vi "Init Frame Grabber.vi"(6 "Frame Grabber":T2="cam1", 8 "Error In":errorcluster, 11 "Frame Grabber Data In":T1={"Camera Session"="", "Frame"=refnum, "AVI Refnum"=refnum, "Codecs"=[], "Frame number"=0, "Tracking File Refnum"=refnum, "Tick Count"=0, "Probe Object"=refnum, "Playback Probe Data"=[], "Rigid Body"={"Position"={"x (mm)"=0.0, "y (mm)"=0.0, "z (mm)"=0.0}, "Orientation"={"Pitch (rad)"=0.0, "Yaw (rad)"=0.0, "Roll (rad)"=0.0}, "Quaternion"={"qx"=0.0, "qy"=0.0, "qz"=0.0, "qw"=0.0}, "Tracked?"=FALSE}, "Total no frames playback"=0, "Video FPS"=0.0, "Camera connected?"=FALSE, "Scene"=refnum, "Cropped Frame"=refnum, "Tracker FPS"=0.0, "Crop ROI"=[], "Presentation Values"=[], "Elapsed time (ms)"=0, "Camera frames playback"=0, "Refnums"={"Live Refnum"=refnum, "Record Refnum"=refnum, "Recording Settings Refnum"=refnum, "Playback Refnum"=refnum, "Frame Slider Refnum"=refnum, "Pause Refnum"=refnum, "Home Refnum"=refnum, "Crop Refnum"=refnum, "Clear Crop Refnum"=refnum, "stop refnum"=refnum, "Playback Rate Refnum"=refnum, "Operator Settings Refnums"=refnum, "Presentation Refnum"=refnum, "Gestation Refnum"=refnum, "Connection Settings Refnum"=refnum, "Crop Time Frame Slider Refnum"=refnum, "Cancel Save Refnum"=refnum, "Reverse Playback Refnum"=refnum}, "Dimensions"={"Probe Dimensions"={"Probe Width"=0.0, "Probe Depth"=1.0, "Probe Height"=0.0}, "Room Dimensions"={"Room Width"=0.0, "Room Depth"=0.0, "Room Height"=0.0}}, "Playback Data As Strings"=[], "Cropped Tracking File Refnum"=refnum, "Cropped AVI Refnum"=refnum, "Header"=[], "Total euclidian distance"=0.0, "Annotation File Path"=path "", "Playback File Path"=path ""}) -> (0 "Error Out":errorcluster={"status"=TRUE, "code"=1088, "source"="Property Node (arg 2) in NI_3D Picture Control.lvlib:Create Box.vi->Create 3D Shapes.vi->Init Frame Grabber.vi->Main.vi"}, 1 "Codec Names":string[](array[string])=["Cinepak Codec by Radius", "Intel IYUV codec", "Microsoft Video 1", "FF Video Codec 1 (FFV1) (NI Vision)", "Motion JPEG (NI Vision)", "Y800 Uncompressed Grey Scale (NI Vision)", "YUV 4:2:0 Planar (NI Vision)"], 2 "Frame Grabber Connected?":bool, 3 "Frame Grabber Data Out":T1={"Camera Session"="", "Frame"=refnum, "AVI Refnum"=refnum, "Codecs"=[], "Frame number"=0, "Tracking File Refnum"=refnum, "Tick Count"=0, "Probe Object"=refnum, "Playback Probe Data"=[], "Rigid Body"={"Position"={"x (mm)"=0.0, "y (mm)"=0.0, "z (mm)"=0.0}, "Orientation"={"Pitch (rad)"=0.0, "Yaw (rad)"=0.0, "Roll (rad)"=0.0}, "Quaternion"={"qx"=0.0, "qy"=0.0, "qz"=0.0, "qw"=0.0}, "Tracked?"=FALSE}, "Total no frames playback"=0, "Video FPS"=0.0, "Camera connected?"=FALSE, "Scene"=refnum, "Cropped Frame"=refnum, "Tracker FPS"=0.0, "Crop ROI"=[], "Presentation Values"=[], "Elapsed time (ms)"=0, "Camera frames playback"=0, "Refnums"={"Live Refnum"=refnum, "Record Refnum"=refnum, "Recording Settings Refnum"=refnum, "Playback Refnum"=refnum, "Frame Slider Refnum"=refnum, "Pause Refnum"=refnum, "Home Refnum"=refnum, "Crop Refnum"=refnum, "Clear Crop Refnum"=refnum, "stop refnum"=refnum, "Playback Rate Refnum"=refnum, "Operator Settings Refnums"=refnum, "Presentation Refnum"=refnum, "Gestation Refnum"=refnum, "Connection Settings Refnum"=refnum, "Crop Time Frame Slider Refnum"=refnum, "Cancel Save Refnum"=refnum, "Reverse Playback Refnum"=refnum}, "Dimensions"={"Probe Dimensions"={"Probe Width"=0.0, "Probe Depth"=1.0, "Probe Height"=0.0}, "Room Dimensions"={"Room Width"=0.0, "Room Depth"=0.0, "Room Height"=0.0}}, "Playback Data As Strings"=[], "Cropped Tracking File Refnum"=refnum, "Cropped AVI Refnum"=refnum, "Header"=[], "Total euclidian distance"=0.0, "Annotation File Path"=path "", "Playback File Path"=path ""}, 4 "Image Out":T3)   [LabVIEW 2017]
uses:
  <vilib>/userdefined/High Color/IMAQdx.ctl
  Controls/Frame Grabber Data.ctl
  <vilib>/vision/Image Controls.llb/IMAQ Image.ctl
  <vilib>/vision/Avi.llb/IMAQ AVI2 Refnum.ctl
  Controls/Rigid Body Info.ctl
  Controls/Position.ctl
  Controls/Orientation.ctl
  Controls/Refnums.ctl
  Controls/Recording Settings.ctl
  Controls/Operator Settings.ctl
  Controls/Operator.ctl
  Controls/Dimensions.ctl
  Controls/Room Dimensions.ctl
  <vilib>/vision/driver/IMAQdx.llb/IMAQdx Camera Control Mode.ctl
  <vilib>/vision/driver/NI_Vision_Acquisition_Software.lvlib
  <vilib>/vision/NI_Vision_Development_Module.lvlib
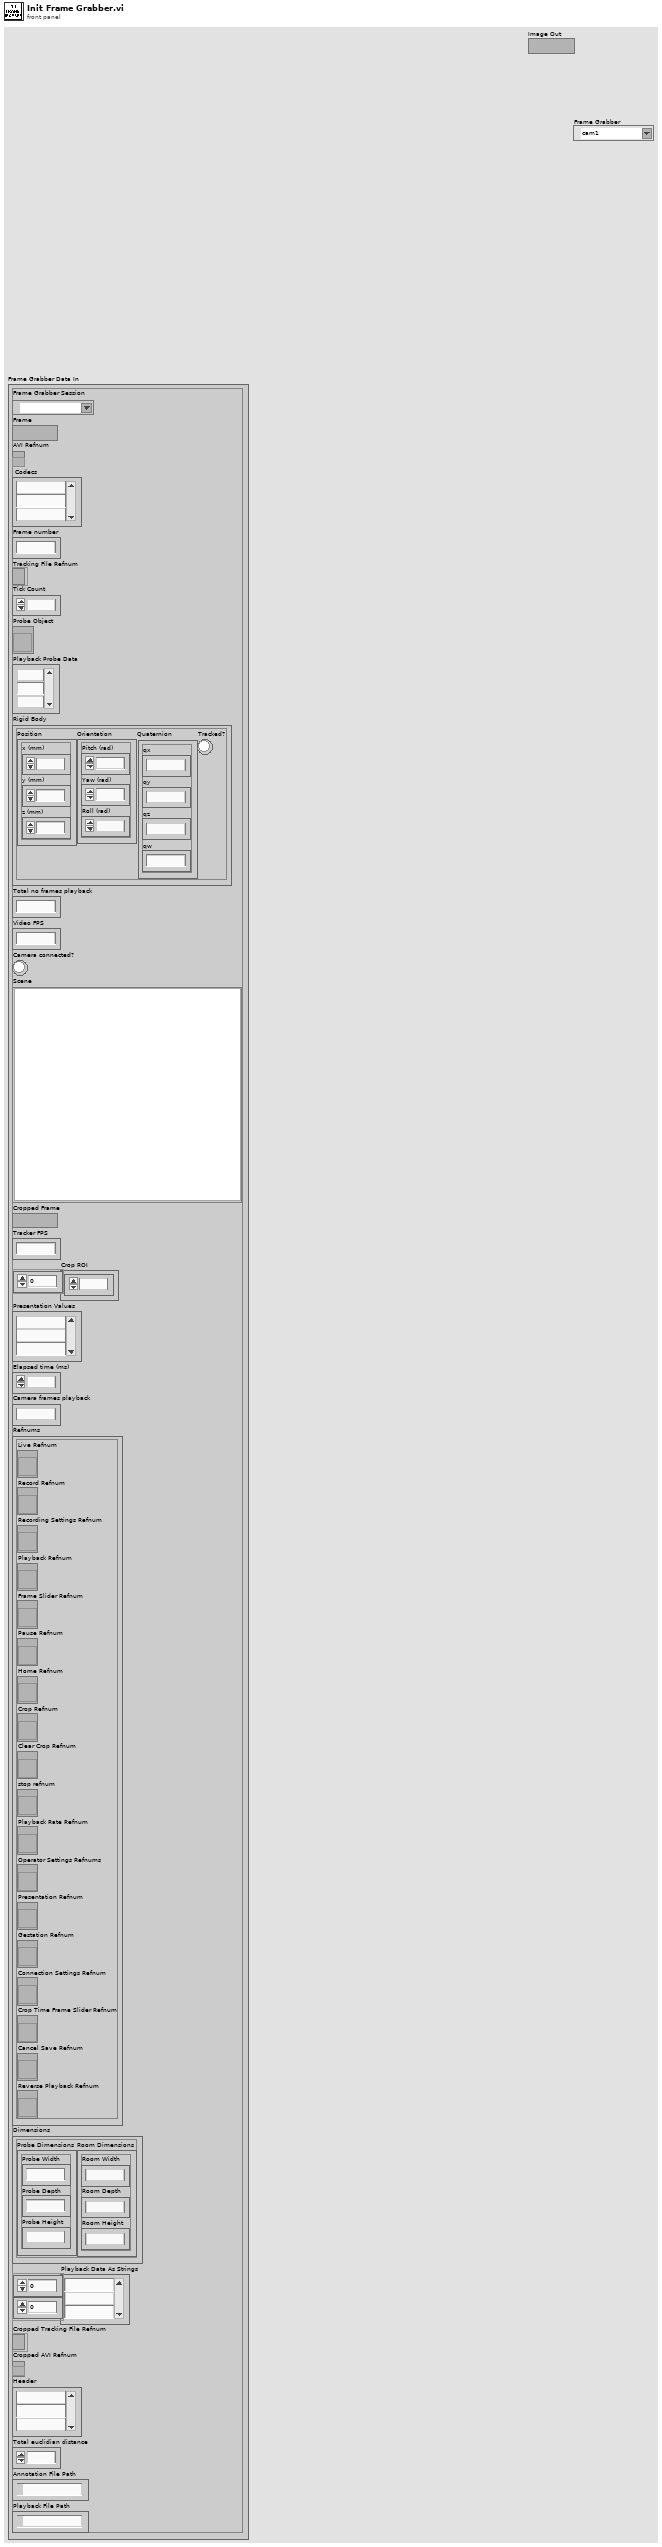
[diagram p1: front panel]
types:
  T1 = typedef "Frame Grabber Data.ctl" = cluster{"Camera Session":T2, "Frame":T3, "AVI Refnum":T4, "Codecs":string[], "Frame number":u32, "Tracking File Refnum":refnum<file>, "Tick Count":u32, "Probe Object":refnum<vi>, "Playback Probe Data":dbl[][], "Rigid Body":T5, "Total no frames playback":i32, "Video FPS":dbl, "Camera connected?":bool, "Scene":refnum<vi>, "Cropped Frame":T3, "Tracker FPS":dbl, "Crop ROI":i32[], "Presentation Values":string[], "Elapsed time (ms)":u32, "Camera frames playback":u32, "Refnums":T8, "Dimensions":T9, "Playback Data As Strings":string[][], "Cropped Tracking File Refnum":refnum<file>, "Cropped AVI Refnum":T4, "Header":string[], "Total euclidian distance":dbl, "Annotation File Path":path, "Playback File Path":path}
  T2 = typedef "IMAQdx.ctl" = refnum<k21>
  T3 = typedef "IMAQ Image.ctl" = refnum<image>
  T4 = typedef "IMAQ AVI2 Refnum.ctl" = refnum<k20>
  T5 = typedef "Rigid Body Info.ctl" = cluster{"Position":T6, "Orientation":T7, "Quaternion":cluster{"qx":sgl, "qy":sgl, "qz":sgl, "qw":sgl}, "Tracked?":bool}
  T6 = typedef "Position.ctl" = cluster{"x (mm)":sgl, "y (mm)":sgl, "z (mm)":sgl}
  T7 = typedef "Orientation.ctl" = cluster{"Pitch (rad)":sgl, "Yaw (rad)":sgl, "Roll (rad)":sgl}
  T8 = typedef "Refnums.ctl" = cluster{"Live Refnum":refnum<vi>, "Record Refnum":refnum<vi>, "Recording Settings Refnum":refnum<vi>, "Playback Refnum":refnum<vi>, "Frame Slider Refnum":refnum<vi>, "Pause Refnum":refnum<vi>, "Home Refnum":refnum<vi>, "Crop Refnum":refnum<vi>, "Clear Crop Refnum":refnum<vi>, "stop refnum":refnum<vi>, "Playback Rate Refnum":refnum<vi>, "Operator Settings Refnums":refnum<vi>, "Presentation Refnum":refnum<vi>, "Gestation Refnum":refnum<vi>, "Connection Settings Refnum":refnum<vi>, "Crop Time Frame Slider Refnum":refnum<vi>, "Cancel Save Refnum":refnum<vi>, "Reverse Playback Refnum":refnum<vi>}
  T9 = typedef "Dimensions.ctl" = cluster{"Probe Dimensions":cluster{"Probe Width":sgl, "Probe Depth":sgl, "Probe Height":sgl}, "Room Dimensions":T10}
  T10 = typedef "Room Dimensions.ctl" = cluster{"Room Width":dbl, "Room Depth":dbl, "Room Height":dbl}
  T11 = typedef "NI_Vision_Acquisition_Software.lvlib/IMAQdx Camera Control Mode.ctl" = enum32{"Controller", "Listener"}
  T12 = typedef "Image Type" = u32
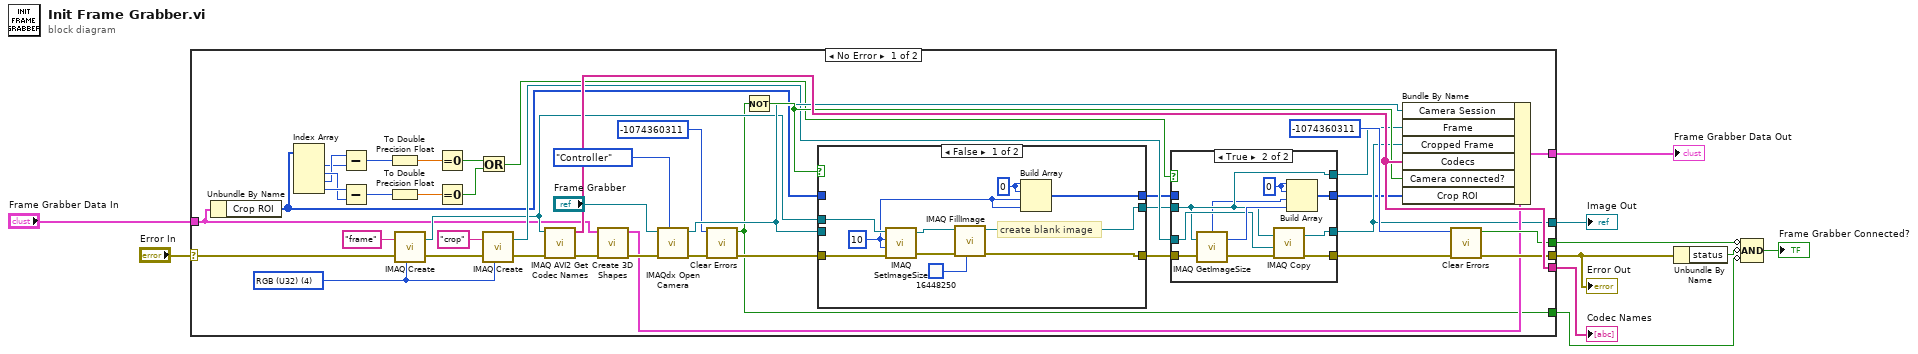
[diagram p0: block diagram]
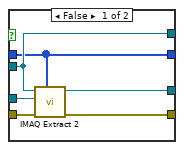
[diagram p2: hidden frame]
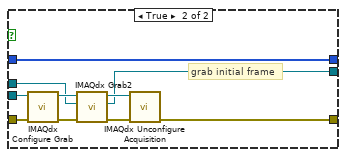
[diagram p3: hidden frame]
diagram:
  n1 = case shown="No Error" "Error In" {
    selector: "Error In" -> [w48 w91]
    tunnel: [w53 _] -> w4
    tunnel: [w45 w91] -> w9
    tunnel: [w51 _] -> w8
    tunnel: [w44 _] -> w6
    tunnel: [w24 _] -> w3
    tunnel: [w13 _] -> w2
    tunnel: "Frame Grabber Data In" -> [w12 _]
    frame No Error {
      w41 = T12 4 items=["Grayscale (U8)", "Grayscale (I16)", "Grayscale (SGL)", "Complex (CSG)", "RGB (U32)", "HSL (U32)", "RGB (U64)", "Grayscale (U16)"] ("Image Type")
      n2 = Unbundle By Name(w12) -> ("Crop ROI"=w11:i32[])
      n3 = Index Array(array=w11) -> (element #1=w19:i32, element #2=w21:i32, element #3=w20:i32, element #4=w22:i32)  [unwired: 4 in]
      n4 = Subtract(x=w20, y=w19) -> (x-y=w36:i32)
      n5 = Subtract(x=w22, y=w21) -> (x-y=w35:i32)
      n6 = To Double Precision Float(number=w36) -> (double precision float=w29:dbl)
      n7 = To Double Precision Float(number=w35) -> (double precision float=w28:dbl)
      n8 = call "IMAQ Create"("Image Name"="frame", "Image Type"=w41, "error in (no error)"=w48) -> ("New Image"=w26:T3, "error out"=w40:errorcluster)  [unwired: 2 in]
      n9 = Equal To 0?(x=w29) -> (x = 0?=w33:bool)
      n10 = Equal To 0?(x=w28) -> (x = 0?=w34:bool)
      n11 = Or(x=w33, y=w34) -> (x .or. y?=w32:bool)
      n12 = call "IMAQ Create"("Image Name"="crop", "Image Type"=w41, "error in (no error)"=w40) -> ("New Image"=w27:T3, "error out"=w39:errorcluster)  [unwired: 2 in]
      n13 = call "IMAQ AVI2 Get Codec Names"("error in (no error)"=w39, "Image"=w26) -> ("error out"=w49:errorcluster, "Codec Names"=w51:string[])  [unwired: 8 in]
      n14 = call "Create 3D Shapes.vi"("error in (no error)"=w49, "Frame Grabber Data In"=w12) -> ("error out"=w47:errorcluster, "Frame Grabber Data Out"=w43:T1)  [unwired: 8 in]
      n15 = call <vilib>:"IMAQdx Open Camera.vi"("Camera Control Mode"=IMAQdx_Camera_Control_Mode."Controller", "error in"=w47, "Session In"="Frame Grabber") -> ("error out"=w15:errorcluster, "Session Out"=w37:T2)  [unwired: 7 in]
      n16 = call <vilib>:"Clear Errors.vi"("error in (no error)"=w15, "specific error code to clear (0: all)"=-1074360311) -> ("error out"=w14:errorcluster, "specific error cleared?"=w13:bool)  [unwired: 4 in]
      n17 = Not(x=w13) -> (.not. x?=w38:bool)
      n18 = case shown="False" w38 {
        tunnel: w14 -> [w80 w87]
        tunnel: [w78 w86] -> w31
        tunnel: w37 -> [_ w85]
        tunnel: w26 -> [w77 w83]
        tunnel: [w75 w82] -> w25
        tunnel: w11 -> [_ w81]
        tunnel: [w73 w81] -> w17
        frame False {
          w72 = 0 ("element")
          w71 = 10 ("X Resolution")
          # "create blank image"
          n19 = call "IMAQ SetImageSize"("error in (no error)"=w80, "Y Resolution"=w71, "X Resolution"=w71, "Image"=w77) -> ("error out"=w79:errorcluster, "Image Out"=w76:T3)  [unwired: 1 in]
          n20 = call "IMAQ FillImage"("Color Pixel Value"=u32 16448250, "error in (no error)"=w79, "Image"=w76) -> ("error out"=w78:errorcluster, "Image Out"=w75:T3)  [unwired: 7 in]
          n21 = Build Array(w72, w72, w71, w71) -> (w73:i32[])
        }
        frame True {
          # "grab initial frame"
          n22 = call <vilib>:"IMAQdx Configure Grab.vi"("error in"=w87, "Session In"=w85) -> ("error out"=w88:errorcluster, "Session Out"=w90:T2)  [unwired: 8 in]
          n23 = call <vilib>:"IMAQdx Grab2.vi"("error in"=w88, "Image In"=w83, "Session In"=w90) -> ("error out"=w89:errorcluster, "Image Out"=w82:T3, "Session Out"=w84:T2)  [unwired: 5 in, 1 out]
          n24 = call <vilib>:"IMAQdx Unconfigure Acquisition.vi"("error in"=w89, "Session In"=w84) -> ("error out"=w86:errorcluster)  [unwired: 8 in, 1 out]
        }
      }
      n25 = case shown="True" w32 {
        tunnel: w25 -> [w56 w65]
        tunnel: w31 -> [w59 w69]
        tunnel: [w58 w64] -> w30
        tunnel: w27 -> [w60 w68]
        tunnel: w17 -> [w55 _]
        tunnel: [w56 w65] -> w23
        tunnel: [w57 w66] -> w24
        tunnel: [w55 w63] -> w18
        frame False {
          n26 = call "IMAQ Extract 2"("Optional Rectangle"=w55, "error in (no error)"=w59, "Image Dst"=w60, "Image Src"=w56) -> ("error out"=w58:errorcluster, "Image Dst Out"=w57:T3)  [unwired: 6 in]
        }
        frame True {
          w61 = 0 ("element")
          n27 = call "IMAQ GetImageSize"("Image"=w65, "error in (no error)"=w69) -> ("Y Resolution"=w70:i32, "X Resolution"=w62:i32, "error out"=w67:errorcluster)  [unwired: 2 in]
          n28 = call "IMAQ Copy"("error in (no error)"=w67, "Image Dst"=w68, "Image Src"=w65) -> ("error out"=w64:errorcluster, "Image Dst Out"=w66:T3)  [unwired: 3 in]
          n29 = Build Array(w61, w61, w62, w70) -> (w63:i32[])
        }
      }
      n30 = Bundle By Name(cluster=w43, "Camera Session"=w37, "Frame"=w23, "Cropped Frame"=w24, "Codecs"=w51, "Camera connected?"=w38, "Crop ROI"=w18) -> (w53:T1)
      n31 = call <vilib>:"Clear Errors.vi"("error in (no error)"=w30, "specific error code to clear (0: all)"=-1074360311) -> ("error out"=w45:errorcluster, "specific error cleared?"=w44:bool)  [unwired: 4 in]
    }
    frame Error {
    }
  }
  "Error Out" <- w9
  "Codec Names" <- w8
  "Frame Grabber Data Out" <- w4
  "Image Out" <- w3
  n32 = Unbundle By Name(w9) -> ("status"=w7:bool)
  n33 = Compound Arithmetic op=AND(invert w6, invert w7, invert w2) -> (→"Frame Grabber Connected?":bool)
